vi "PhidgetGetChannelClass.vi"(0 "error in (no error)":errorcluster, 3 "Device In":u64) -> (7 "error out":errorcluster, 9 "Channel Class":u32(ring) items=["PHIDCHCLASS_NOTHING", "PHIDCHCLASS_ACCELEROMETER", "PHIDCHCLASS_CURRENTINPUT", "PHIDCHCLASS_DATAADAPTER", "PHIDCHCLASS_DCMOTOR", "PHIDCHCLASS_DIGITALINPUT", "PHIDCHCLASS_DIGITALOUTPUT", "PHIDCHCLASS_DISTANCESENSOR", "PHIDCHCLASS_ENCODER", "PHIDCHCLASS_FREQUENCYCOUNTER", "PHIDCHCLASS_GPS", "PHIDCHCLASS_LCD", "PHIDCHCLASS_GYROSCOPE", "PHIDCHCLASS_HUB", "PHIDCHCLASS_HUMANINPUT", "PHIDCHCLASS_HUMIDITYSENSOR", "PHIDCHCLASS_IR", "PHIDCHCLASS_LIGHTSENSOR", "PHIDCHCLASS_MAGNETOMETER", "PHIDCHCLASS_MESHDONGLE", "PHIDCHCLASS_POWERGUARD", "PHIDCHCLASS_PRESSURESENSOR", "PHIDCHCLASS_RCSERVO", "PHIDCHCLASS_RESISTANCEINPUT", "PHIDCHCLASS_RFID", "PHIDCHCLASS_SOUNDSENSOR", "PHIDCHCLASS_SPATIAL", "PHIDCHCLASS_STEPPER", "PHIDCHCLASS_TEMPERATURESENSOR", "PHIDCHCLASS_VOLTAGEINPUT", "PHIDCHCLASS_VOLTAGEOUTPUT", "PHIDCHCLASS_VOLTAGERATIOINPUT", "", "", "PHIDCHCLASS_MOTORPOSITIONCONTROLLER", "PHIDCHCLASS_BLDCMOTOR", "PHIDCHCLASS_DICTIONARY"], 10 "Device Out":u64)   [LabVIEW 2012, in "Phidget Common.lvlib"]
doc: "${ChannelClass:Header}"
uses:
  <instrlib>/Phidgets/Phidget Common/Phidget Common.lvlib
  phidget22.dll
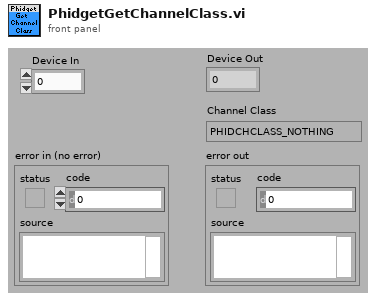
[diagram p1: front panel]
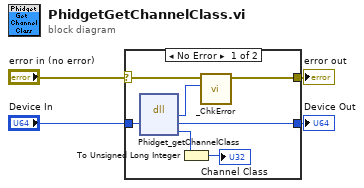
[diagram p0: block diagram]
diagram:
  n1 = case shown="No Error" "error in (no error)" {
    selector: "error in (no error)" -> [w11 w13]
    tunnel: [w10 w13] -> w3
    tunnel: "Device In" -> [w8 w12]
    tunnel: [w9 w12] -> w1
    frame No Error {
      n2 = dll-call lib="phidget22.dll" fn="Phidget_getChannelClass"("phid"=w8) -> ("return type"=w7:i32, "phid"=w9:u64, "Channel"=w5:i32)  [unwired: 4 in, 2 out]
      n3 = To Unsigned Long Integer(number=w5) -> (unsigned 32bit integer=→"Channel Class":u32)
      n4 = call <instrlib>:"_ChkError.vi"("Return Code"=w7, "error in (no error)"=w11) -> ("error out"=w10:errorcluster)  [unwired: 9 in]
    }
    frame Error {
    }
  }
  "error out" <- w3
  "Device Out" <- w1
